vi "Spectrum Single Shot Demo.vi"() -> ()   [LabVIEW 2012]
uses:
  LabVIEW/user.lib/SpectralRadar.llb/set Spectrum Output.vi
  LabVIEW/user.lib/SpectralRadar.llb/display Data 1D.vi
  LabVIEW/user.lib/SpectralRadar.llb/OCT Device.lvclass
  LabVIEW/user.lib/SpectralRadar.llb/Processing.lvclass
  LabVIEW/user.lib/SpectralRadar.llb/Raw Data.lvclass
  LabVIEW/user.lib/SpectralRadar.llb/Data.lvclass
panel:
  in  "NumberOfSpectra":i32=10 min=1 step=1
  out "Spectrum":dbl[](graph)
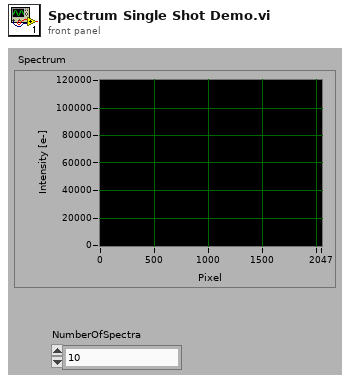
[diagram p1: front panel]
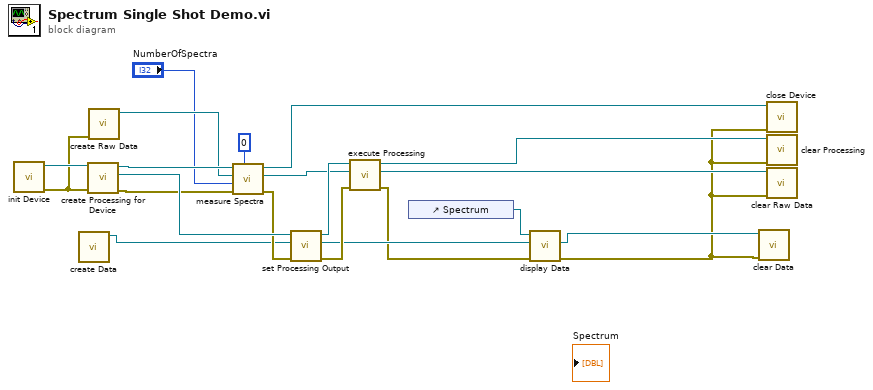
[diagram p0: block diagram]
diagram:
  n1 = call "init Device.vi"() -> ("error out"=w16:errorcluster, "OCTDevice"=w17:refnum<class "OCT Device.lvclass">)  [unwired: 6 in]
  n2 = call "create Data.vi"() -> ("Data"=w4:refnum<class "Data.lvclass">)  [unwired: 6 in, 1 out]
  n3 = call "create Processing for Device.vi"("error in (no error)"=w16, "OCTDevice"=w17) -> ("error out"=w18:errorcluster, "Processing"=w20:refnum<class "Processing.lvclass">, "OCTDevice"=w21:refnum<class "OCT Device.lvclass">)  [unwired: 3 in]
  n4 = call "create Raw Data.vi"("error in (no error)"=w16) -> ("Raw Data"=w19:refnum<class "Raw Data.lvclass">)  [unwired: 5 in, 1 out]
  n5 = call "measure Spectra.vi"("Camera #"=0, "error in (no error)"=w18, "NumberOfSpectra"="NumberOfSpectra", "Raw Data"=w19, "OCTDevice"=w21) -> ("error out"=w12:errorcluster, "Raw Data"=w10:refnum<class "Raw Data.lvclass">, "OCTDevice"=w15:refnum<class "OCT Device.lvclass">)  [unwired: 1 in]
  n6 = call-poly "set Processing Output.vi"("error in (no error)"=w12, "Data"=w4, "Processing"=w20) -> ("error out"=w9:errorcluster, "Data"=w8:refnum<class "Data.lvclass">, "Processing"=w11:refnum<class "Processing.lvclass">)  [unwired: 2 in]
  n7 = call "execute Processing.vi"("error in (no error)"=w9, "Raw Data"=w10, "Processing"=w11) -> ("error out"=w6:errorcluster, "Raw Data"=w13:refnum<class "Raw Data.lvclass">, "Processing"=w14:refnum<class "Processing.lvclass">)  [unwired: 2 in]
  n8 = control-ref of="Spectrum"() -> (w7:refnum<vi>)
  n9 = call-poly "display Data.vi"("error in (no error)"=w6, "Data in"=w8, "WFGraph Refnum"=w7) -> ("error out"=w2:errorcluster, "Data out"=w3:refnum<class "Data.lvclass">)  [unwired: 2 in, 1 out]
  n10 = call "clear Data.vi"("error in (no error)"=w2, "Data"=w3) -> ()  [unwired: 5 in, 1 out]
  n11 = call "close Device.vi"("error in (no error)"=w2, "OCTDevice"=w15) -> ()  [unwired: 5 in, 1 out]
  n12 = call "clear Processing.vi"("error in (no error)"=w2, "Processing"=w14) -> ()  [unwired: 5 in, 1 out]
  n13 = call "clear Raw Data.vi"("error in (no error)"=w2, "Raw Data"=w13) -> ()  [unwired: 5 in, 1 out]
